vi "from string array.vi"(8 "error in (no error)":errorcluster, 9 "String Array":string[][](array[string]), 10 "version":string, 11 "Increment configuration in":refnum<class "Increment configuration.lvclass">) -> (0 "error out":errorcluster, 3 "Increment configuration out":refnum<class "Increment configuration.lvclass">)   [LabVIEW 2015, in "Increment configuration.lvclass"]
uses:
  Increment configuration.lvclass
  Increment configuration.lvclass/Increment configuration.ctl
  Write Lines.vi
  Get Line Name.vi
  <vilib>/NI/Tag Bus Module Framework/module configuration/FindDuplicate.vi
  <vilib>/Utility/error.llb/Error Cluster From Error Code.vi
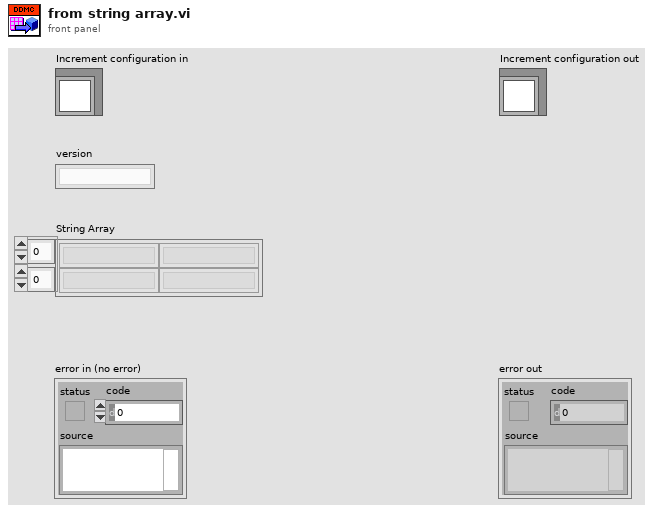
[diagram p1: front panel]
types:
  T1 = typedef "Increment configuration.lvclass/Line.ctl" = cluster{"Name":string, "channel in":refnum<class "TBM channel.lvclass">, "channel out":refnum<class "TBM channel.lvclass">}
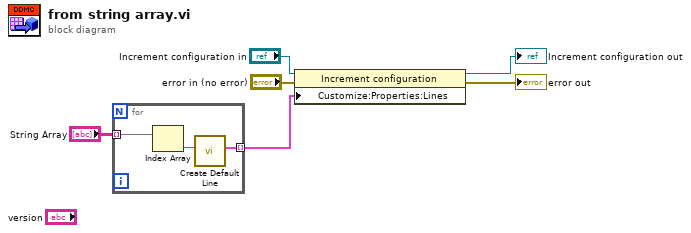
[diagram p0: block diagram]
diagram:
  n1 = for {
    tunnel: "String Array" -> [w9] mode=indexing
    tunnel: [w7] -> w1 mode=indexing
    n2 = Index Array(array=w9) -> (element=w8:string)  [unwired: 1 in]
    n3 = call "Create Default Line.vi"("Line Name"=w8) -> ("output cluster"=w7:T1)  [unwired: 10 in]
  }
  n4 = property class="Increment configuration"(reference="Increment configuration in", error in="error in (no error)", "Customize:Properties:Lines"=w1) -> (reference out=→"Increment configuration out":refnum<class "Increment configuration.lvclass">, error out=→"error out":errorcluster)
